vi "SRV_Sensor View Tab GUI.vi"(10 "SRV In":refnum<k5>, 11 "Sensors Config File Path":path) -> (0 "error out":errorcluster)   [LabVIEW 2009]
doc: "A Producer-Consumer two-loop state machine template. This template uses the LPD Command Queues to drive its execution.\n\nThere are several advantages such as:\n- convenient error state control\n- the ability to pass data between states/loops/VIs via a variant\n- command history which is extremely valuable in troubleshooting when an error occurs\n\n\nAuthor: Mike Schultz\n\nLogicPD, Inc\nwww.logicpd.com"
uses:
  SRV_Sensor View refs.ctl
  SRV_Sensor Config Cluster.ctl
  SRV_Sensor Analog-Digital.ctl
  SRV_Sensor Sampling Mode.ctl
  SRV_Sensor View Config Cluster.ctl
  SRV_Sensors Names.ctl
  SRV_Sensor PicoC Shared Var Type.ctl
  SRV_Sensor Config-Command Cluster.ctl
  Support/SRV_Command-Data Queue Data Type.ctl
  SRV_Sensor-Value Cluster.ctl
  <vilib>/Utility/error.llb/DialogType.ctl
panel:
  out "Overflow Indicator":bool
  out "# elements in queue":i32
  out "Command":string
  in  "Poll":bool
  in  "Edit_Boolean 32":bool
  out "Boolean 32":bool
  in  "Edit_Boolean 31":bool
  out "Boolean 31":bool
  in  "Edit_Boolean 30":bool
  out "Boolean 30":bool
  in  "Edit_Boolean 29":bool
  out "Boolean 29":bool
  in  "Edit_Boolean 28":bool
  out "Boolean 28":bool
  in  "Edit_Boolean 27":bool
  out "Boolean 27":bool
  in  "Edit_Boolean 26":bool
  out "Boolean 26":bool
  in  "Edit_Boolean 25":bool
  out "Boolean 25":bool
  in  "Edit_Boolean 24":bool
  out "Boolean 24":bool
  in  "Edit_Boolean 23":bool
  out "Boolean 23":bool
  in  "Edit_Boolean 22":bool
  out "Boolean 22":bool
  in  "Edit_Boolean 21":bool
  out "Boolean 21":bool
  in  "Edit_Boolean 20":bool
  out "Boolean 20":bool
  in  "Edit_Boolean 19":bool
  out "Boolean 19":bool
  in  "Edit_Boolean 18":bool
  out "Boolean 18":bool
  in  "Edit_Boolean 17":bool
  out "Boolean 17":bool
  in  "Edit_Boolean 16":bool
  out "Boolean 16":bool
  in  "Edit_Boolean 15":bool
  out "Boolean 15":bool
  in  "Edit_Boolean 14":bool
  out "Boolean 14":bool
  in  "Edit_Boolean 13":bool
  out "Boolean 13":bool
  in  "Edit_Boolean 12":bool
  out "Boolean 12":bool
  in  "Edit_Boolean 11":bool
  out "Boolean 11":bool
  in  "Edit_Boolean 10":bool
  out "Boolean 10":bool
  in  "Edit_Boolean 09":bool
  out "Boolean 09":bool
  in  "Edit_Boolean 08":bool
  out "Boolean 08":bool
  in  "Edit_Boolean 07":bool
  out "Boolean 07":bool
  in  "Edit_Boolean 06":bool
  out "Boolean 06":bool
  in  "Edit_Boolean 05":bool
  out "Boolean 05":bool
  in  "Edit_Boolean 04":bool
  out "Boolean 04":bool
  in  "Edit_Boolean 03":bool
  out "Boolean 03":bool
  in  "Edit_Boolean 02":bool
  out "Boolean 02":bool
  in  "Edit_Boolean 01":bool
  out "Boolean 01":bool
  in  "Edit_Numeric 08":bool
  out "Numeric 08":dbl
  in  "Edit_Numeric 07":bool
  out "Numeric 07":dbl
  in  "Edit_Numeric 06":bool
  out "Numeric 06":dbl
  in  "Edit_Numeric 05":bool
  out "Numeric 05":dbl
  in  "Edit_Numeric 04":bool
  out "Numeric 04":dbl
  in  "Edit_Numeric 03":bool
  out "Numeric 03":dbl
  in  "Edit_Numeric 02":bool
  out "Numeric 02":dbl
  in  "Edit_Numeric 01":bool
  out "Numeric 01":dbl
  in  "Edit_Meter 04":bool
  out "Meter 04":dbl(knob) scale=-1.0..0.0
  in  "Edit_Meter 03":bool
  out "Meter 03":dbl(knob) scale=-1.0..0.0
  in  "Edit_Meter 02":bool
  out "Meter 02":dbl(knob) caption="6" scale=-1.0..0.0
  in  "Edit_Meter 01":bool
  out "Meter 01":dbl(knob) caption="5" scale=-1.0..0.0
  in  "Edit_Gauge 04":bool
  out "Gauge 04":dbl(knob) caption="4" scale=-1.0..0.0
  in  "Edit_Gauge 03":bool
  out "Gauge 03":dbl(knob) caption="3" scale=-1.0..0.0
  in  "Edit_Gauge 02":bool
  out "Gauge 02":dbl(knob) caption="2" scale=-1.0..0.0
  in  "Edit_Gauge 01":bool
  out "Gauge 01":dbl(knob) caption="1" scale=-1.0..0.0 scale format="%#.3g"
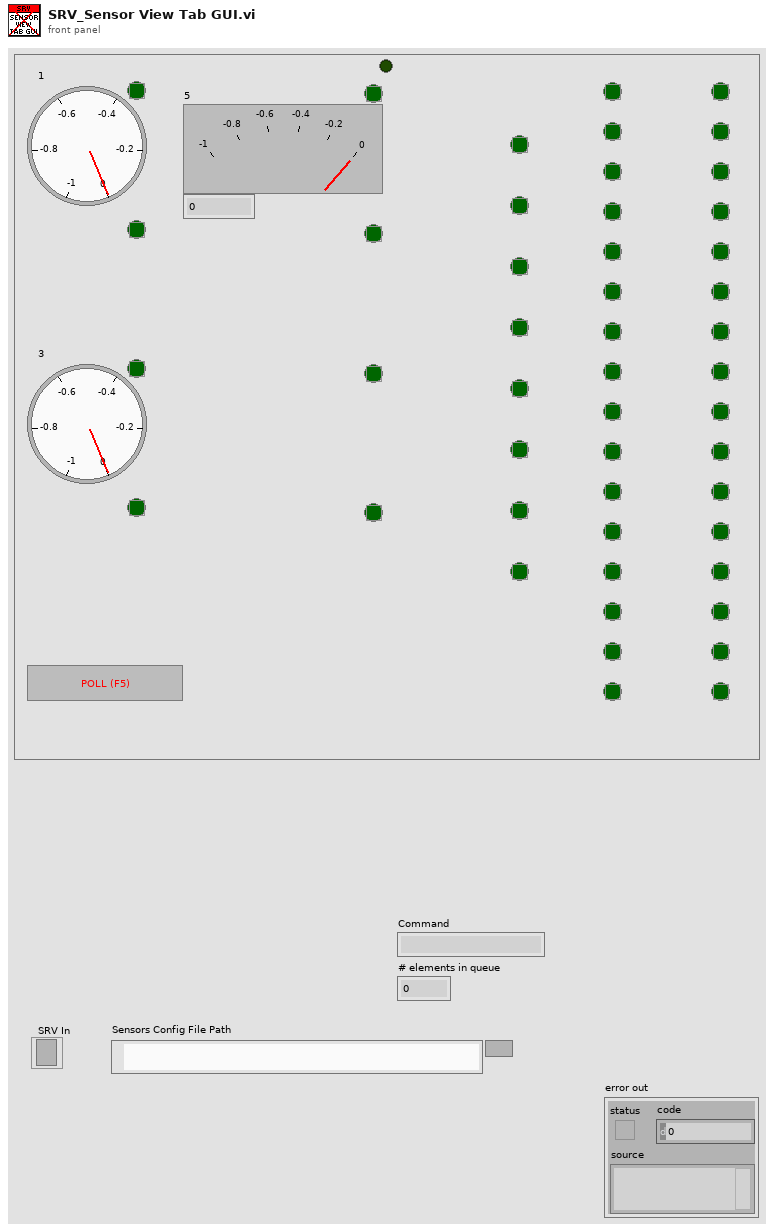
[diagram p1: front panel]
types:
  T1 = typedef "SRV_Command-Data Queue Data Type.ctl" = cluster{"Command":string, "Data":variant}
  T2 = typedef "SRV_Sensor View refs.ctl" = cluster{"Knob refs":refnum<vi>[], "Numeric refs":refnum<vi>[], "Boolean refs":refnum<vi>[]}
  T3 = typedef "SRV_Sensor Config Cluster.ctl" = cluster{"Name":string, "A/D":T4, "I2C Address":u8, "Register":u8, "Channel":u8, "Digital Mask":u8, "Units":string, "Sampling Mode":T5, "Sample Period (ms)":u32, "Formula":string, "Sensor View Config":T6, "Active":bool, "PicoC Shared Var Type":T8, "Index":u8, "Stream Multiple?":bool, "Index End":u8}
  T4 = typedef "SRV_Sensor Analog-Digital.ctl" = enum16{"Analog", "Digital", "RCMx1 Analog", "PicoC Shared"}
  T5 = typedef "SRV_Sensor Sampling Mode.ctl" = enum16{"Polled", "Streaming"}
  T6 = typedef "SRV_Sensor View Config Cluster.ctl" = cluster{"Sensor Name":T7, "Minimum":dbl, "Maximum":dbl}
  T7 = typedef "SRV_Sensors Names.ctl" = enum16{"Gauge 01", "Gauge 02", "Gauge 03", "Gauge 04", "Meter 01", "Meter 02", "Meter 03", "Meter 04", "Numeric 01", "Numeric 02", "Numeric 03", "Numeric 04", "Numeric 05", "Numeric 06", "Numeric 07", "Numeric 08", "Boolean 01", "Boolean 02", "Boolean 03", "Boolean 04", "Boolean 05", "Boolean 06", "Boolean 07", "Boolean 08", "Boolean 09", "Boolean 10", "Boolean 11", "Boolean 12", "Boolean 13", "Boolean 14", "Boolean 15", "Boolean 16", "Boolean 17", "Boolean 18", "Boolean 19", "Boolean 20", "Boolean 21", "Boolean 22", "Boolean 23", "Boolean 24", "Boolean 25", "Boolean 26", "Boolean 27", "Boolean 28", "Boolean 29", "Boolean 30", "Boolean 31", "Boolean 32"}
  T8 = typedef "SRV_Sensor PicoC Shared Var Type.ctl" = enum16{"String", "Integer", "Float"}
  T9 = typedef "SRV_Sensor Config-Command Cluster.ctl" = cluster{"Sensor Config":T3, "Command":string, "Constant Command":string}
  T10 = cluster{"user event":refnum<user-event>, "Version":string, "Sensor View refs":T2, "This VI ref":refnum<vi>, "Sensors Config File Path":path, "Sensors Config":T3[], "SRV ref":refnum<k5>, "Streaming Cfg-Cmds":T9[], "Polled Cfg-Cmds":T9[], "Off Cfg-Cmds":T9[], "Streaming Constant Commands":string[], "Polled Constant Commands":string[]}
  T11 = typedef "SRV_Sensor-Value Cluster.ctl" = cluster{"Sensor Name":T7, "Value":dbl}
  T12 = typedef "DialogType.ctl" = u16
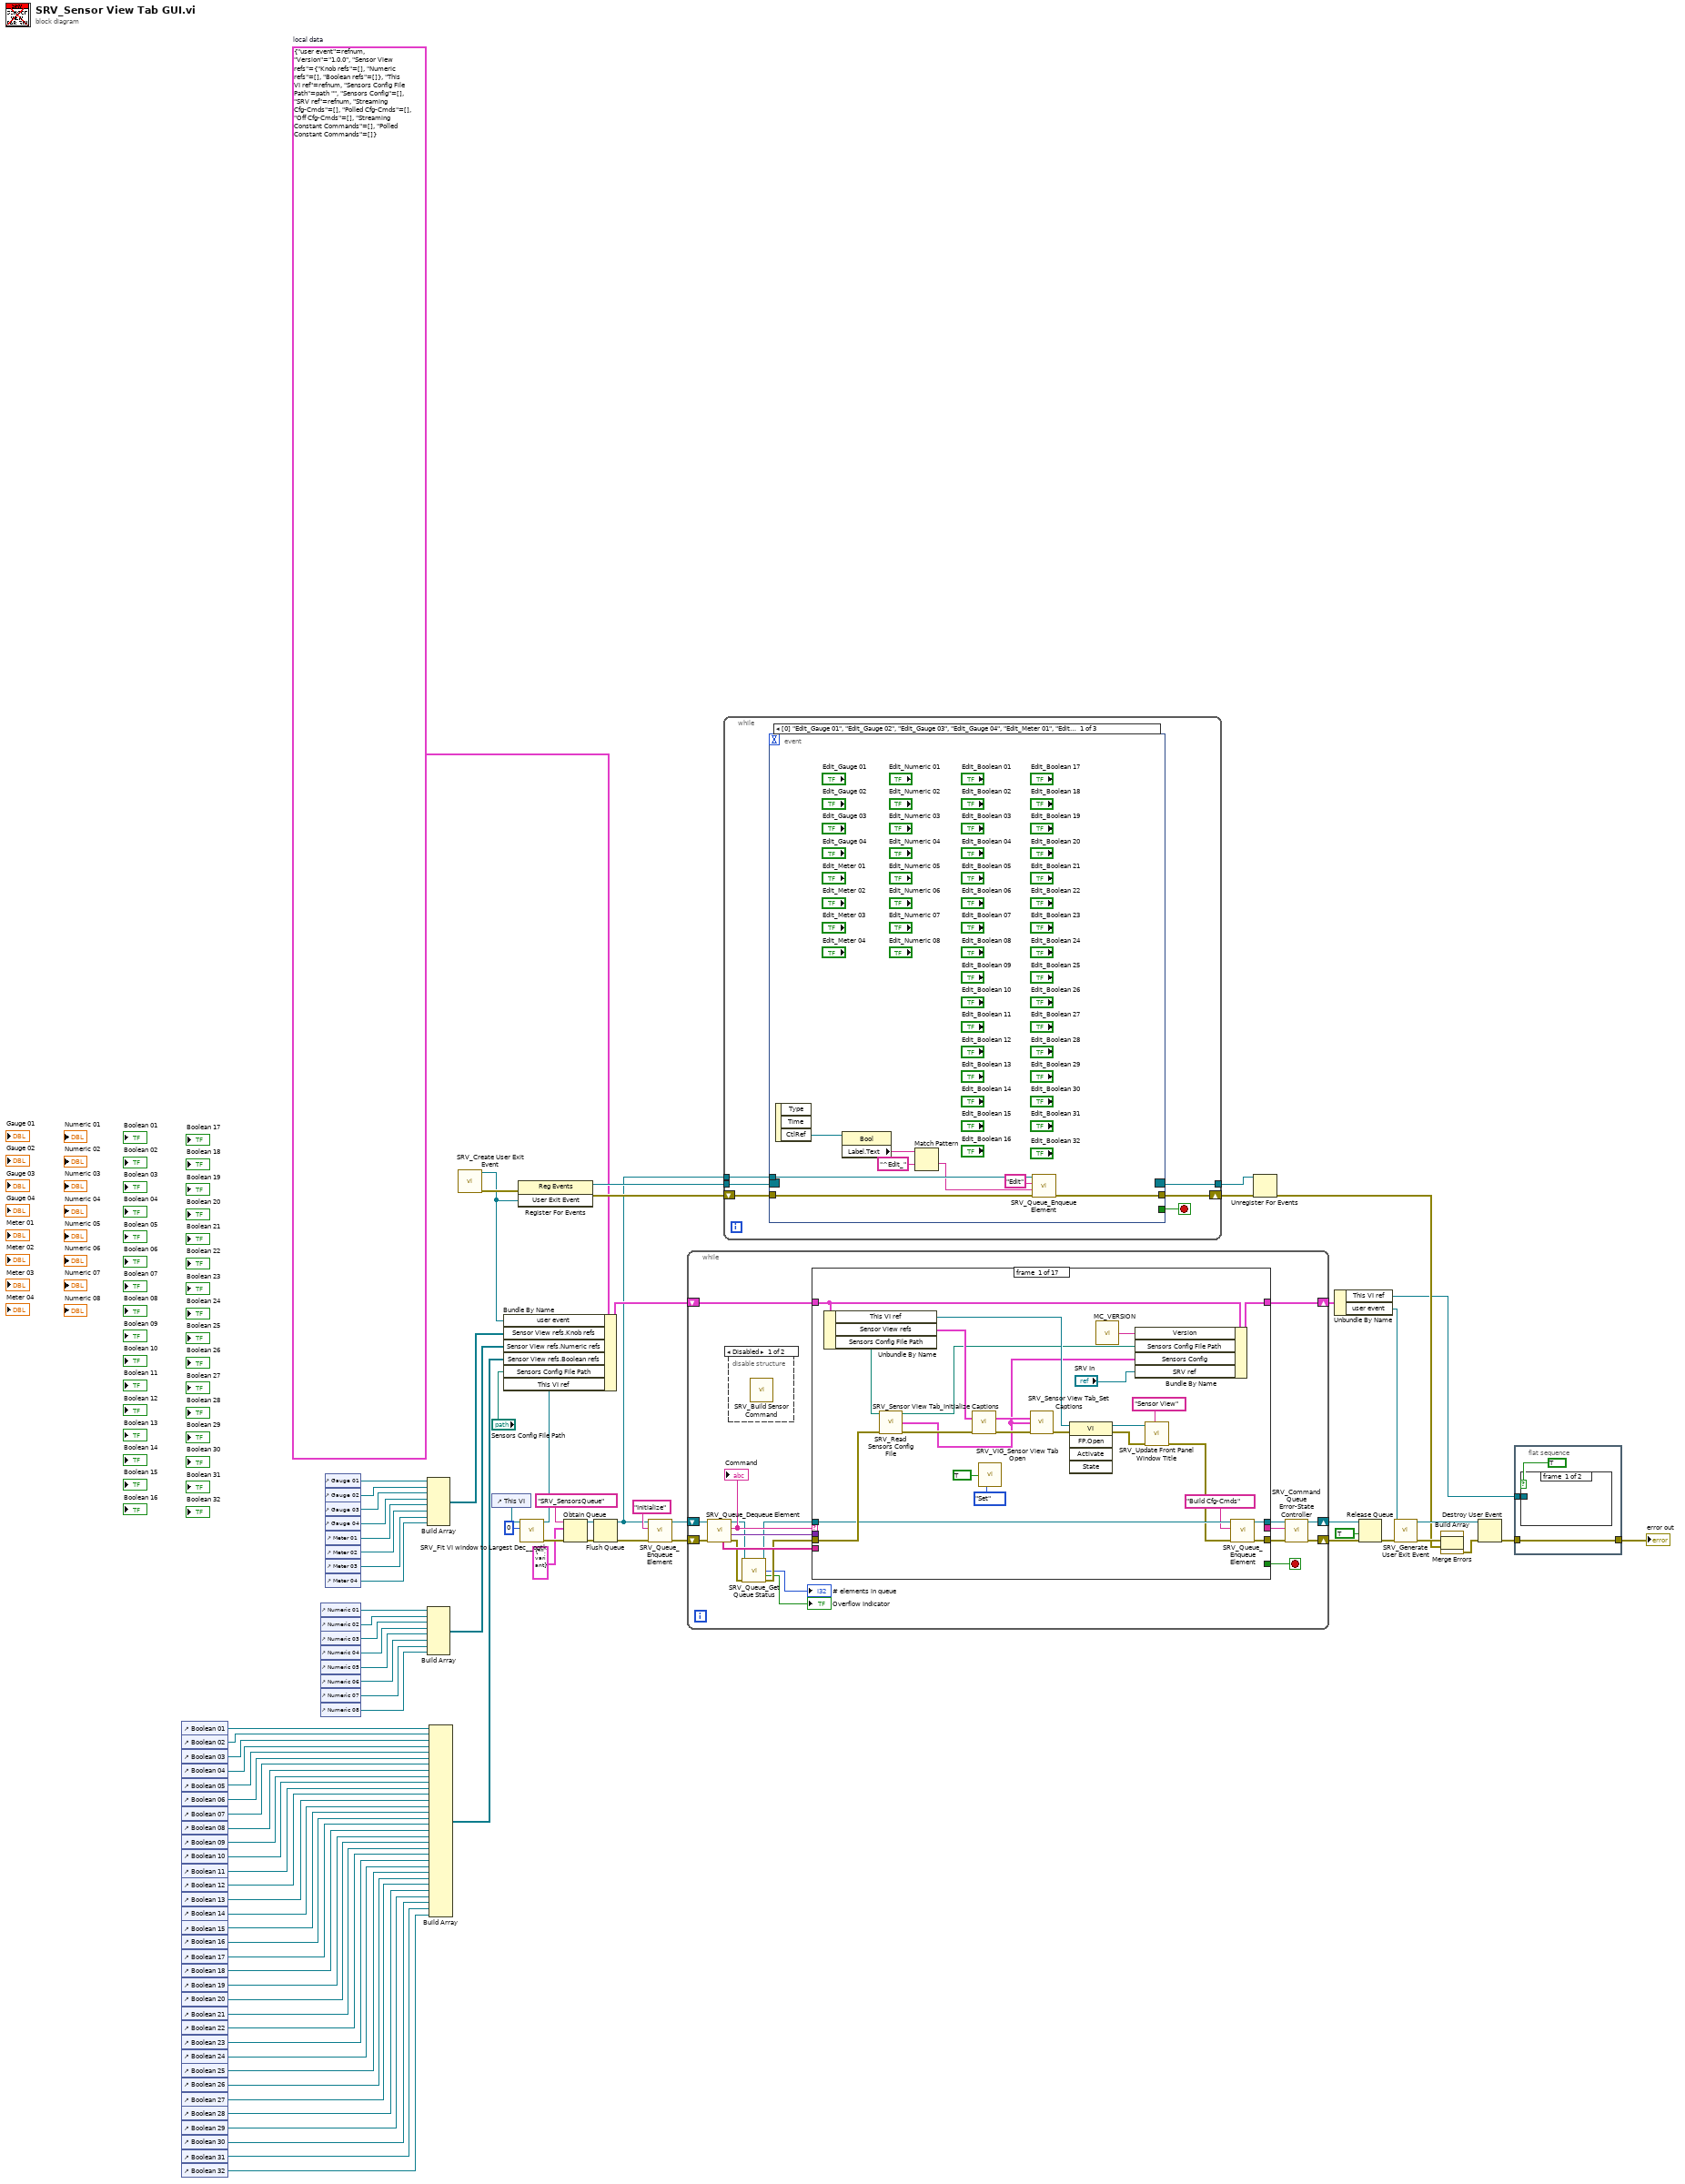
[diagram p0: block diagram]
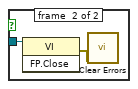
[diagram p2: hidden frame]
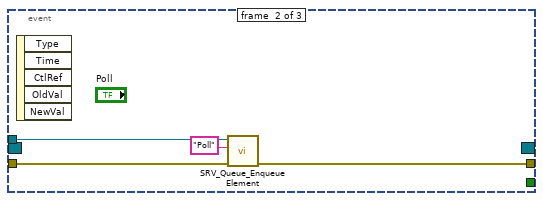
[diagram p3: hidden frame]
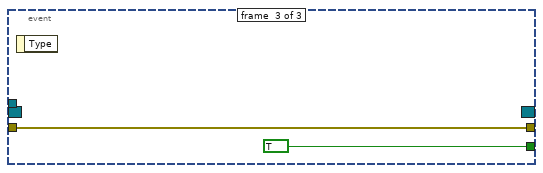
[diagram p4: hidden frame]
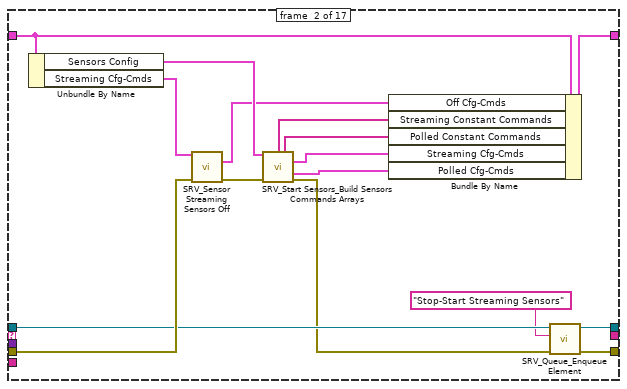
[diagram p6: hidden frame]
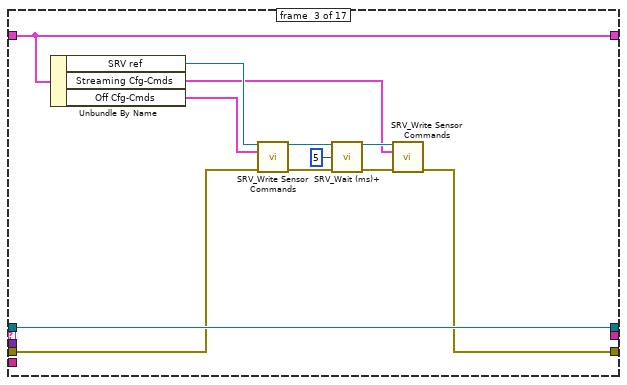
[diagram p7: hidden frame]
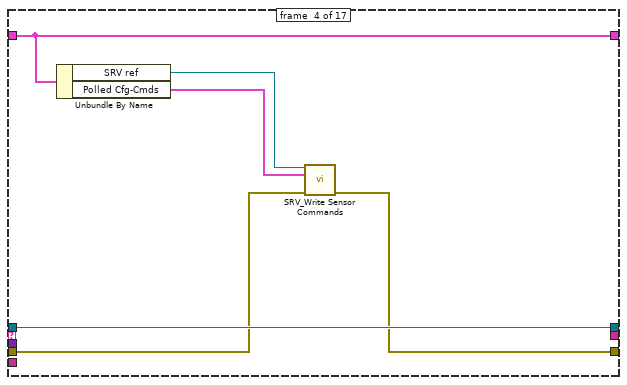
[diagram p8: hidden frame]
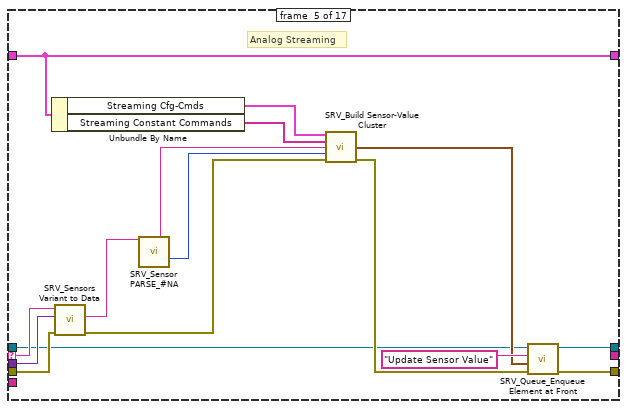
[diagram p9: hidden frame]
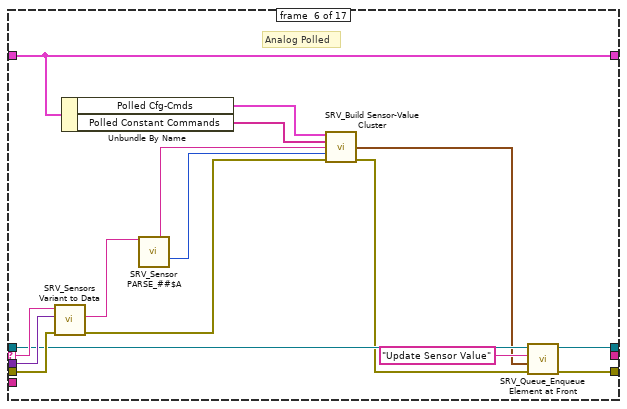
[diagram p10: hidden frame]
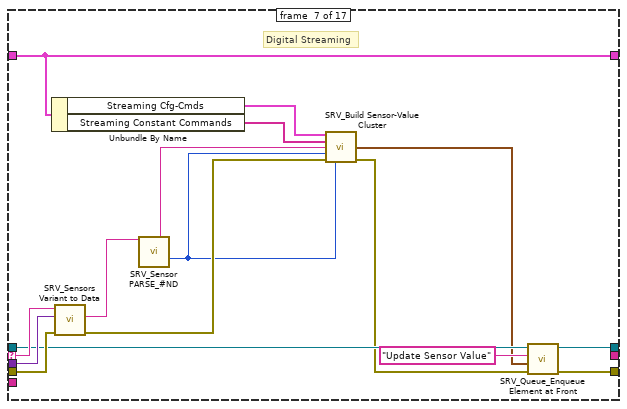
[diagram p11: hidden frame]
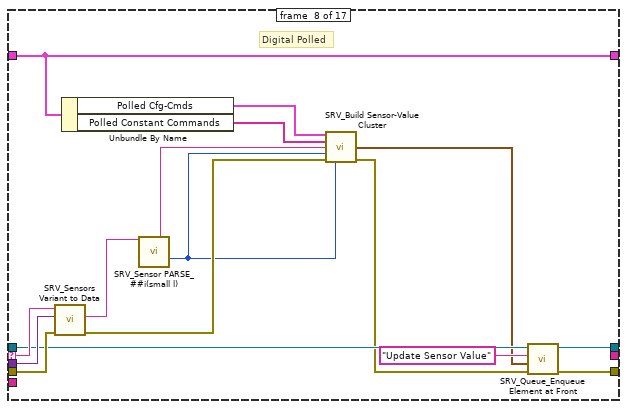
[diagram p12: hidden frame]
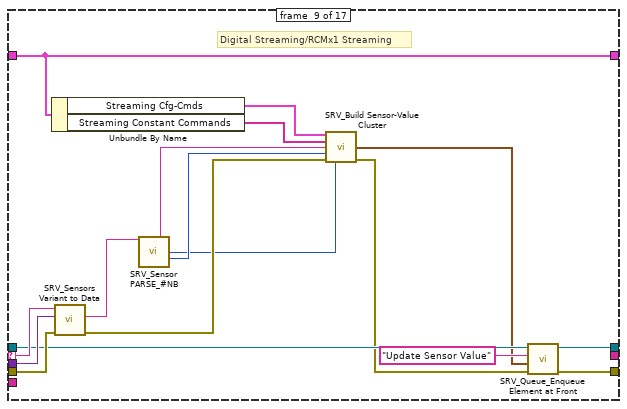
[diagram p13: hidden frame]
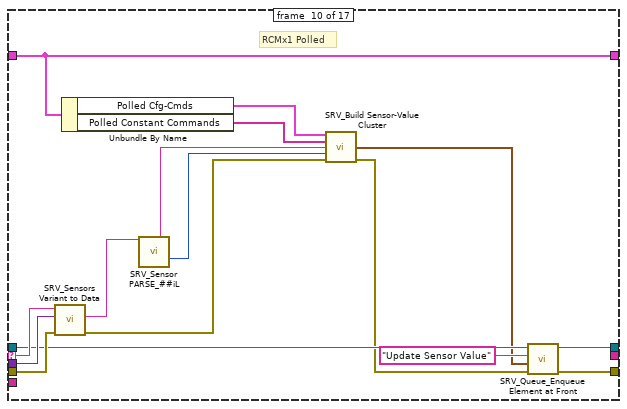
[diagram p14: hidden frame]
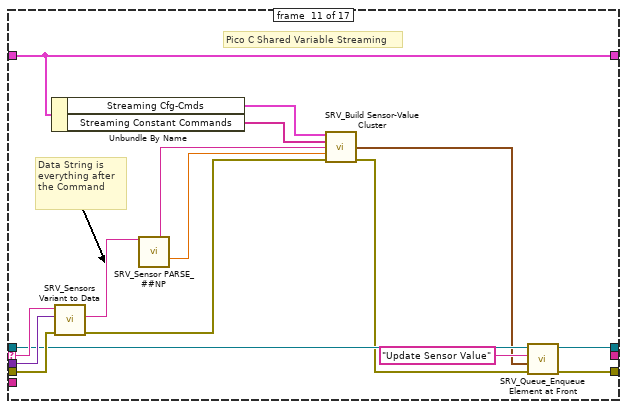
[diagram p15: hidden frame]
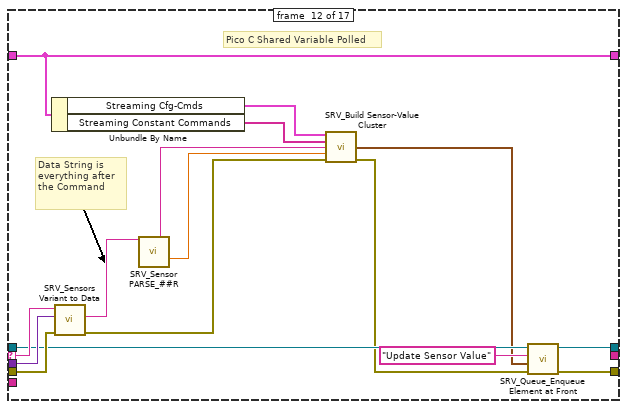
[diagram p16: hidden frame]
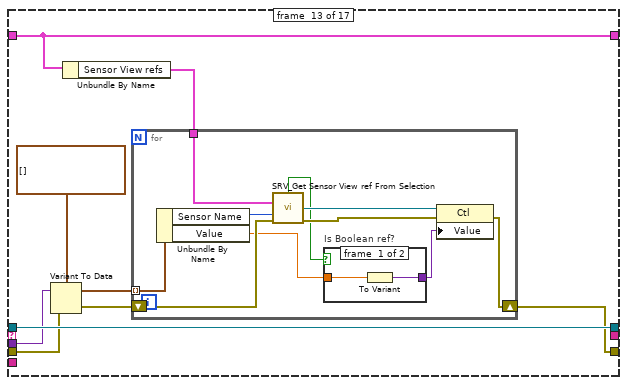
[diagram p17: hidden frame]
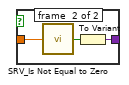
[diagram p18: hidden frame]
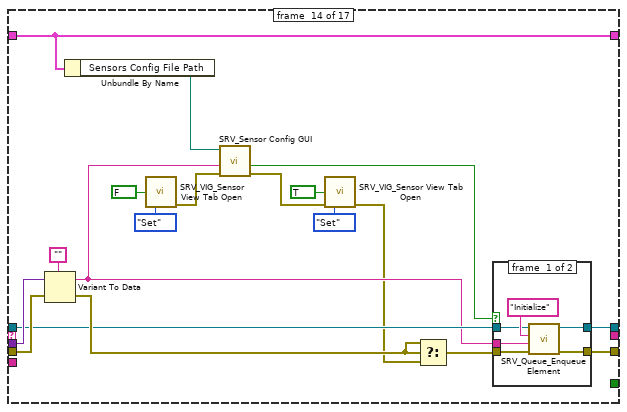
[diagram p19: hidden frame]
diagram:
  w81 = T10 {"user event"=refnum, "Version"="1.0.0", "Sensor View refs"={"Knob refs"=[], "Numeric refs"=[], "Boolean refs"=[]}, "This VI ref"=refnum, "Sensors Config File Path"=path "", "Sensors Config"=[], "SRV ref"=refnum, "Streaming Cfg-Cmds"=[], "Polled Cfg-Cmds"=[], "Off Cfg-Cmds"=[], "Streaming Constant Commands"=[], "Polled Constant Commands"=[]}  # local data
  n1 = control-ref of="Boolean 01"() -> (w48:refnum<vi>)
  n2 = control-ref of="Boolean 02"() -> (w47:refnum<vi>)
  n3 = control-ref of="Boolean 03"() -> (w46:refnum<vi>)
  n4 = control-ref of="Boolean 04"() -> (w45:refnum<vi>)
  n5 = control-ref of="Boolean 05"() -> (w44:refnum<vi>)
  n6 = control-ref of="Boolean 06"() -> (w43:refnum<vi>)
  n7 = control-ref of="Boolean 07"() -> (w42:refnum<vi>)
  n8 = control-ref of="Boolean 08"() -> (w41:refnum<vi>)
  n9 = control-ref of="Boolean 09"() -> (w40:refnum<vi>)
  n10 = control-ref of="Boolean 10"() -> (w39:refnum<vi>)
  n11 = control-ref of="Boolean 11"() -> (w38:refnum<vi>)
  n12 = control-ref of="Boolean 12"() -> (w37:refnum<vi>)
  n13 = control-ref of="Boolean 13"() -> (w36:refnum<vi>)
  n14 = control-ref of="Boolean 14"() -> (w35:refnum<vi>)
  n15 = control-ref of="Boolean 15"() -> (w34:refnum<vi>)
  n16 = control-ref of="Boolean 16"() -> (w33:refnum<vi>)
  n17 = control-ref of="Boolean 17"() -> (w32:refnum<vi>)
  n18 = control-ref of="Boolean 18"() -> (w31:refnum<vi>)
  n19 = control-ref of="Boolean 19"() -> (w30:refnum<vi>)
  n20 = control-ref of="Boolean 20"() -> (w29:refnum<vi>)
  n21 = control-ref of="Boolean 21"() -> (w28:refnum<vi>)
  n22 = control-ref of="Boolean 22"() -> (w27:refnum<vi>)
  n23 = control-ref of="Boolean 23"() -> (w26:refnum<vi>)
  n24 = control-ref of="Boolean 24"() -> (w25:refnum<vi>)
  n25 = control-ref of="Boolean 25"() -> (w24:refnum<vi>)
  n26 = control-ref of="Boolean 26"() -> (w23:refnum<vi>)
  n27 = control-ref of="Boolean 27"() -> (w22:refnum<vi>)
  n28 = control-ref of="Boolean 28"() -> (w21:refnum<vi>)
  n29 = control-ref of="Boolean 29"() -> (w20:refnum<vi>)
  n30 = control-ref of="Boolean 30"() -> (w19:refnum<vi>)
  n31 = control-ref of="Boolean 31"() -> (w18:refnum<vi>)
  n32 = control-ref of="Boolean 32"() -> (w17:refnum<vi>)
  n33 = control-ref of="Numeric 01"() -> (w56:refnum<vi>)
  n34 = control-ref of="Numeric 02"() -> (w55:refnum<vi>)
  n35 = control-ref of="Numeric 03"() -> (w54:refnum<vi>)
  n36 = control-ref of="Numeric 04"() -> (w53:refnum<vi>)
  n37 = control-ref of="Numeric 05"() -> (w52:refnum<vi>)
  n38 = control-ref of="Numeric 06"() -> (w51:refnum<vi>)
  n39 = control-ref of="Numeric 07"() -> (w50:refnum<vi>)
  n40 = control-ref of="Numeric 08"() -> (w49:refnum<vi>)
  n41 = control-ref of="Gauge 01"() -> (w64:refnum<vi>)
  n42 = control-ref of="Gauge 02"() -> (w63:refnum<vi>)
  n43 = control-ref of="Gauge 03"() -> (w62:refnum<vi>)
  n44 = control-ref of="Gauge 04"() -> (w61:refnum<vi>)
  n45 = control-ref of="Meter 01"() -> (w60:refnum<vi>)
  n46 = control-ref of="Meter 02"() -> (w59:refnum<vi>)
  n47 = control-ref of="Meter 03"() -> (w58:refnum<vi>)
  n48 = control-ref of="Meter 04"() -> (w57:refnum<vi>)
  n49 = Build Array(w64, w63, w62, w61, w60, w59, w58, w57) -> (w11:refnum<vi>[])
  n50 = Build Array(w56, w55, w54, w53, w52, w51, w50, w49) -> (w12:refnum<vi>[])
  n51 = Build Array(w48, w47, w46, w45, w44, w43, w42, w41, w40, w39, w38, w37, w36, w35, w34, w33, w32, w31, w30, w29, w28, w27, w26, w25, w24, w23, w22, w21, w20, w19, w18, w17) -> (w13:refnum<vi>[])
  n52 = call "SRV_Create User Exit Event.vi"() -> ("error out"=w72:errorcluster, "User Exit Event"=w71:refnum<user-event>)  [unwired: 10 in]
  n53 = control-ref of="This VI"() -> (w2:refnum<vi>)
  n54 = register-events(error in=w72, w71) -> (reference out=w87:refnum<event-registration>, error out=w86:errorcluster)  [unwired: 1 in]
  n55 = call "SRV_Fit VI window to Largest Dec__ogtk.vi"("border spacing (2 px)"=0, "VI Ref (calling VI)"=w2) -> ("error out"=w67:errorcluster, "dup VI Ref"=w10:refnum<vi>)  [unwired: 4 in]
  n56 = Bundle By Name(cluster=w81, "user event"=w71, "Sensor View refs.Knob refs"=w11, "Sensor View refs.Numeric refs"=w12, "Sensor View refs.Boolean refs"=w13, "Sensors Config File Path"="Sensors Config File Path", "This VI ref"=w10) -> (w80:T10)
  n57 = Obtain Queue(name (unnamed)="SRV_SensorsQueue", element data type=T1 {"Command"="", "Data"=variant} ("Queue Data Type"), error in (no error)=w67) -> (queue out=w4:refnum<queue>, error out=w6:errorcluster)  [unwired: 2 in, 1 out]
  n58 = Flush Queue(queue=w4, error in (no error)=w6) -> (queue out=w3:refnum<queue>, error out=w5:errorcluster)  [unwired: 1 out]
  n59 = call "SRV_Queue_Enqueue Element.vi"("error in (no error)"=w5, "Command"="Initialize", "Command-Data Queue"=w3) -> ("error out"=w65:errorcluster, "Command-Data Queue out"=w68:refnum<queue>)  [unwired: 6 in, 1 out]
  n60 = while {
    shift-right: [w102] -> w83
    shift-left: w65 -> [w106]
    shift-right: [w100] -> w82
    shift-left: w68 -> [w105]
    shift-right: [w94] -> w79
    shift-left: w80 -> [w95]
    stop <- w96 stop-if-true
    n61 = call "SRV_Queue_Dequeue Element.vi"("error in (no error)"=w106, "Command-Data Queue"=w105) -> ("error out"=w93:errorcluster, "Data"=w99:variant, "Command"=w104:string, "Command-Data Queue out"=w91:refnum<queue>, "Command History"=w98:string[])  [unwired: 4 in, 1 out]
    "Command" <- w104
    n62 = disable-structure shown="Disabled" {
      frame #0 {
        n63 = call "SRV_Build Sensor Command.vi"() -> ()  [unwired: 9 in, 7 out]
      }
      frame #1 {
      }
    }
    n64 = call "SRV_Queue_Get Queue Status.vi"("Command-Data Queue"=w91, "error in (no error)"=w93) -> ("Command-Data Queue out"=w90:refnum<queue>, "# elements in queue"=→"# elements in queue":i32, "Overflow Indicator"=→"Overflow Indicator":bool, "error out"=w92:errorcluster)  [unwired: 10 in]
    n65 = case shown="\"Initialize\"" w104 {
      selector: w104 -> [_ _ _ _ w178 w194 w210 w226 w243 w259 w275 w291 _ _ w348 _ _]
      tunnel: w92 -> [w129 w140 w155 w159 w165 w193 w209 w225 w242 w258 w274 w290 w300 w335 w346 w355 w362]
      tunnel: [w116 w135 w150 w158 w169 w182 w199 w215 w232 w247 w263 w279 w294 w328 w345 w352 w361] -> w103
      tunnel: w90 -> [w118 w137 w156 w163 w164 w185 w202 w218 w235 w250 w266 w282 w301 w326 w350 w359 w372]
      tunnel: [w117 w136 w156 w163 w171 w184 w201 w217 w234 w249 w265 w281 w301 w327 w350 w359 w372] -> w101
      tunnel: w99 -> [_ _ _ _ w179 w195 w211 w227 w244 w260 w276 w292 w299 w333 _ _ _]
      tunnel: w98 -> [_ _ _ _ _ _ _ _ _ _ _ _ _ _ _ w358 _]
      tunnel: [_ _ _ _ _ _ _ _ _ _ _ _ _ _ _ "Exit" ("Error Command") _] -> w97
      tunnel: [_ _ _ _ _ _ _ _ _ _ _ _ _ _ _ _ TRUE] -> w96
      tunnel: w95 -> [w127 w145 w157 w162 w176 w191 w207 w223 w240 w256 w272 w288 w298 w331 w347 w356 w368]
      tunnel: [w130 w144 w157 w162 w176 w191 w207 w223 w240 w256 w272 w288 w298 w331 w347 w356 w368] -> w94
      frame #0 {
        n66 = Unbundle By Name(w127) -> ("This VI ref"=w123:refnum<vi>, "Sensor View refs"=w126:T2, "Sensors Config File Path"=w120:path)
        n67 = call "SRV_Read Sensors Config File.vi"("Sensors Config File Path"=w120, "error in (no error)"=w129) -> ("Sensors Config File Path out"=w121:path, "Sensors Config"=w119:T3[], "error out"=w128:errorcluster)  [unwired: 10 in, 1 out]
        n68 = call "SRV_Sensor View Tab_Initialize Captions.vi"("Sensor View refs"=w126, "error in (no error)"=w128) -> ("Sensor View refs dup"=w124:T2, "error out"=w125:errorcluster)  [unwired: 12 in]
        n69 = call "SRV_VIG_Sensor View Tab Open.vi"("Sensor View Tab Open"=TRUE, "Method (Get)"=enum16{"Get", "Set"}."Set") -> ()  [unwired: 12 in, 2 out]
        n70 = call "SRV_Sensor View Tab_Set Captions.vi"("Sensor View refs"=w124, "Sensors Config"=w119, "error in (no error)"=w125) -> ("error out"=w122:errorcluster)  [unwired: 11 in, 1 out]
        n71 = invoke class="VI" method="FP.Open"(reference=w123, error in=w122) -> (reference out=w111:refnum<vi>, error out=w112:errorcluster)  [unwired: 3 in, 3 out]
        n72 = call "MC_VERSION.vi"() -> ("MC Version"=w113:string)
        n73 = Bundle By Name(cluster=w127, "Version"=w113, "Sensors Config File Path"=w121, "Sensors Config"=w119, "SRV ref"="SRV In") -> (w130:T10)
        n74 = call "SRV_Update Front Panel Window Title.vi"("Window Title Override String"="Sensor View", "error in (no error)"=w112, "VI ref"=w111) -> ("error out"=w110:errorcluster)  [unwired: 7 in, 1 out]
        n75 = call "SRV_Queue_Enqueue Element.vi"("error in (no error)"=w110, "Command"="Build Cfg-Cmds", "Command-Data Queue"=w118) -> ("error out"=w116:errorcluster, "Command-Data Queue out"=w117:refnum<queue>)  [unwired: 6 in, 1 out]
      }
      frame #1 {
        n76 = Unbundle By Name(w145) -> ("Sensors Config"=w146:T3[], "Streaming Cfg-Cmds"=w141:T9[])
        n77 = call "SRV_Sensor Streaming Sensors Off.vi"("Previous Streaming Cfg-Cmds"=w141, "error in (no error)"=w140) -> ("Streaming Cfg-Cmds OFF"=w138:T9[], "error out"=w139:errorcluster)  [unwired: 12 in]
        n78 = call "SRV_Start Sensors_Build Sensors Commands Arrays.vi"("Sensors Config"=w146, "error in (no error)"=w139) -> ("Streaming Constant Commands"=w132:string[], "Polled Constant Commands"=w131:string[], "Active Streaming Cfg-Commands"=w143:T9[], "Active Polled Cfg-Commands"=w142:T9[], "error out"=w134:errorcluster)  [unwired: 9 in]
        n79 = Bundle By Name(cluster=w145, "Off Cfg-Cmds"=w138, "Streaming Constant Commands"=w132, "Polled Constant Commands"=w131, "Streaming Cfg-Cmds"=w143, "Polled Cfg-Cmds"=w142) -> (w144:T10)
        n80 = call "SRV_Queue_Enqueue Element.vi"("error in (no error)"=w134, "Command"="Stop-Start Streaming Sensors", "Command-Data Queue"=w137) -> ("error out"=w135:errorcluster, "Command-Data Queue out"=w136:refnum<queue>)  [unwired: 6 in, 1 out]
      }
      frame #2 {
        n81 = Unbundle By Name(w157) -> ("SRV ref"=w154:refnum<k5>, "Streaming Cfg-Cmds"=w151:T9[], "Off Cfg-Cmds"=w153:T9[])
        n82 = call "SRV_Write Sensor Commands.vi"("SRV In"=w154, "Sensor Cfg-Commands"=w153, "error in (no error)"=w155) -> ("SRV out"=w152:refnum<k5>, "error out"=w149:errorcluster)  [unwired: 11 in]
        n83 = call "SRV_Wait (ms)+.vi"("milliseconds to wait"=u32 5, "error in (no error)"=w149) -> ("error out"=w148:errorcluster)  [unwired: 12 in, 1 out]
        n84 = call "SRV_Write Sensor Commands.vi"("SRV In"=w152, "Sensor Cfg-Commands"=w151, "error in (no error)"=w148) -> ("error out"=w150:errorcluster)  [unwired: 11 in, 1 out]
      }
      frame #3 {
        n85 = Unbundle By Name(w162) -> ("SRV ref"=w160:refnum<k5>, "Polled Cfg-Cmds"=w161:T9[])
        n86 = call "SRV_Write Sensor Commands.vi"("SRV In"=w160, "Sensor Cfg-Commands"=w161, "error in (no error)"=w159) -> ("error out"=w158:errorcluster)  [unwired: 11 in, 1 out]
      }
      frame #4 {
        # "Analog Streaming"
        n87 = Unbundle By Name(w176) -> ("Streaming Cfg-Cmds"=w175:T9[], "Streaming Constant Commands"=w174:string[])
        n88 = call "SRV_Sensors Variant to Data.vi"("error in (no error)"=w165, "Data"=w179, "Command"=w178) -> ("error out"=w166:errorcluster, "Data String"=w177:string)  [unwired: 7 in]
        n89 = call "SRV_Sensor PARSE_#NA.vi"("Return Data"=w177) -> ("Constant Command"=w173:string, "Value"=w172:u16)  [unwired: 13 in]
        n90 = call "SRV_Build Sensor-Value Cluster.vi"("Cfg-Cmds"=w175, "Constant Commands"=w174, "Constant Command"=w173, "Value"=w172, "error in (no error)"=w166) -> ("Array of Sensor-Value Cluster"=w167:T11[], "error out"=w170:errorcluster)  [unwired: 9 in]
        n91 = call "SRV_Queue_Enqueue Element at Front.vi"("error in (no error)"=w170, "Data"=w167, "Command"="Update Sensor Value", "Command-Data Queue"=w164) -> ("error out"=w169:errorcluster, "Command-Data Queue out"=w171:refnum<queue>)  [unwired: 5 in, 1 out]
      }
      frame #5 {
        # "Analog Polled"
        n92 = call "SRV_Sensors Variant to Data.vi"("error in (no error)"=w193, "Data"=w195, "Command"=w194) -> ("error out"=w186:errorcluster, "Data String"=w192:string)  [unwired: 7 in]
        n93 = Unbundle By Name(w191) -> ("Polled Cfg-Cmds"=w190:T9[], "Polled Constant Commands"=w189:string[])
        n94 = call "SRV_Sensor PARSE_##$A.vi"("Return Data"=w192) -> ("Constant Command"=w188:string, "Value"=w187:u16)  [unwired: 13 in]
        n95 = call "SRV_Build Sensor-Value Cluster.vi"("Cfg-Cmds"=w190, "Constant Commands"=w189, "Constant Command"=w188, "Value"=w187, "error in (no error)"=w186) -> ("Array of Sensor-Value Cluster"=w180:T11[], "error out"=w183:errorcluster)  [unwired: 9 in]
        n96 = call "SRV_Queue_Enqueue Element at Front.vi"("error in (no error)"=w183, "Data"=w180, "Command"="Update Sensor Value", "Command-Data Queue"=w185) -> ("error out"=w182:errorcluster, "Command-Data Queue out"=w184:refnum<queue>)  [unwired: 5 in, 1 out]
      }
      frame #6 {
        # "Digital Streaming"
        n97 = Unbundle By Name(w207) -> ("Streaming Cfg-Cmds"=w206:T9[], "Streaming Constant Commands"=w205:string[])
        n98 = call "SRV_Sensors Variant to Data.vi"("error in (no error)"=w209, "Data"=w211, "Command"=w210) -> ("error out"=w203:errorcluster, "Data String"=w208:string)  [unwired: 7 in]
        n99 = call "SRV_Sensor PARSE_#ND.vi"("Return Data"=w208) -> ("Constant Command"=w204:string, "Value"=w196:u8)  [unwired: 13 in]
        n100 = call "SRV_Build Sensor-Value Cluster.vi"("Cfg-Cmds"=w206, "Constant Commands"=w205, "Constant Command"=w204, "Value"=w196, "error in (no error)"=w203, "Value (U8)"=w196) -> ("Array of Sensor-Value Cluster"=w197:T11[], "error out"=w200:errorcluster)  [unwired: 8 in]
        n101 = call "SRV_Queue_Enqueue Element at Front.vi"("error in (no error)"=w200, "Data"=w197, "Command"="Update Sensor Value", "Command-Data Queue"=w202) -> ("error out"=w199:errorcluster, "Command-Data Queue out"=w201:refnum<queue>)  [unwired: 5 in, 1 out]
      }
      frame #7 {
        # "Digital Polled"
        n102 = call "SRV_Sensors Variant to Data.vi"("error in (no error)"=w225, "Data"=w227, "Command"=w226) -> ("error out"=w219:errorcluster, "Data String"=w224:string)  [unwired: 7 in]
        n103 = Unbundle By Name(w223) -> ("Polled Cfg-Cmds"=w222:T9[], "Polled Constant Commands"=w221:string[])
        n104 = call "SRV_Sensor PARSE_##i(small l).vi"("Return Data"=w224) -> ("Constant Command"=w220:string, "Value"=w212:u8)  [unwired: 13 in]
        n105 = call "SRV_Build Sensor-Value Cluster.vi"("Cfg-Cmds"=w222, "Constant Commands"=w221, "Constant Command"=w220, "Value"=w212, "error in (no error)"=w219, "Value (U8)"=w212) -> ("Array of Sensor-Value Cluster"=w213:T11[], "error out"=w216:errorcluster)  [unwired: 8 in]
        n106 = call "SRV_Queue_Enqueue Element at Front.vi"("error in (no error)"=w216, "Data"=w213, "Command"="Update Sensor Value", "Command-Data Queue"=w218) -> ("error out"=w215:errorcluster, "Command-Data Queue out"=w217:refnum<queue>)  [unwired: 5 in, 1 out]
      }
      frame #8 {
        # "Digital Streaming/RCMx1 Streaming"
        n107 = Unbundle By Name(w240) -> ("Streaming Cfg-Cmds"=w239:T9[], "Streaming Constant Commands"=w238:string[])
        n108 = call "SRV_Sensors Variant to Data.vi"("error in (no error)"=w242, "Data"=w244, "Command"=w243) -> ("error out"=w236:errorcluster, "Data String"=w241:string)  [unwired: 7 in]
        n109 = call "SRV_Sensor PARSE_#NB.vi"("Return Data"=w241) -> ("Constant Command"=w237:string, "Value (U8)"=w228:u8, "Value"=w229:u16)  [unwired: 12 in]
        n110 = call "SRV_Build Sensor-Value Cluster.vi"("Cfg-Cmds"=w239, "Constant Commands"=w238, "Constant Command"=w237, "Value"=w229, "error in (no error)"=w236, "Value (U8)"=w228) -> ("Array of Sensor-Value Cluster"=w230:T11[], "error out"=w233:errorcluster)  [unwired: 8 in]
        n111 = call "SRV_Queue_Enqueue Element at Front.vi"("error in (no error)"=w233, "Data"=w230, "Command"="Update Sensor Value", "Command-Data Queue"=w235) -> ("error out"=w232:errorcluster, "Command-Data Queue out"=w234:refnum<queue>)  [unwired: 5 in, 1 out]
      }
      frame #9 {
        # "RCMx1 Polled"
        n112 = call "SRV_Sensors Variant to Data.vi"("error in (no error)"=w258, "Data"=w260, "Command"=w259) -> ("error out"=w251:errorcluster, "Data String"=w257:string)  [unwired: 7 in]
        n113 = Unbundle By Name(w256) -> ("Polled Cfg-Cmds"=w255:T9[], "Polled Constant Commands"=w254:string[])
        n114 = call "SRV_Sensor PARSE_##iL.vi"("Return Data"=w257) -> ("Constant Command"=w253:string, "Value"=w252:u16)  [unwired: 13 in]
        n115 = call "SRV_Build Sensor-Value Cluster.vi"("Cfg-Cmds"=w255, "Constant Commands"=w254, "Constant Command"=w253, "Value"=w252, "error in (no error)"=w251) -> ("Array of Sensor-Value Cluster"=w245:T11[], "error out"=w248:errorcluster)  [unwired: 9 in]
        n116 = call "SRV_Queue_Enqueue Element at Front.vi"("error in (no error)"=w248, "Data"=w245, "Command"="Update Sensor Value", "Command-Data Queue"=w250) -> ("error out"=w247:errorcluster, "Command-Data Queue out"=w249:refnum<queue>)  [unwired: 5 in, 1 out]
      }
      frame #10 {
        # "Data String is everything after the Command"
        # "Pico C Shared Variable Streaming"
        n117 = Unbundle By Name(w272) -> ("Streaming Cfg-Cmds"=w271:T9[], "Streaming Constant Commands"=w270:string[])
        n118 = call "SRV_Sensors Variant to Data.vi"("error in (no error)"=w274, "Data"=w276, "Command"=w275) -> ("error out"=w267:errorcluster, "Data String"=w273:string)  [unwired: 7 in]
        n119 = call "SRV_Sensor PARSE_##NP.vi"("Return Data"=w273) -> ("Constant Command"=w269:string, "Value"=w268:dbl)  [unwired: 13 in]
        n120 = call "SRV_Build Sensor-Value Cluster.vi"("Cfg-Cmds"=w271, "Constant Commands"=w270, "Constant Command"=w269, "Value"=w268, "error in (no error)"=w267) -> ("Array of Sensor-Value Cluster"=w261:T11[], "error out"=w264:errorcluster)  [unwired: 9 in]
        n121 = call "SRV_Queue_Enqueue Element at Front.vi"("error in (no error)"=w264, "Data"=w261, "Command"="Update Sensor Value", "Command-Data Queue"=w266) -> ("error out"=w263:errorcluster, "Command-Data Queue out"=w265:refnum<queue>)  [unwired: 5 in, 1 out]
      }
      frame #11 {
        # "Data String is everything after the Command"
        # "Pico C Shared Variable Polled"
        n122 = Unbundle By Name(w288) -> ("Streaming Cfg-Cmds"=w287:T9[], "Streaming Constant Commands"=w286:string[])
        n123 = call "SRV_Sensors Variant to Data.vi"("error in (no error)"=w290, "Data"=w292, "Command"=w291) -> ("error out"=w283:errorcluster, "Data String"=w289:string)  [unwired: 7 in]
        n124 = call "SRV_Sensor PARSE_##R.vi"("Return Data"=w289) -> ("Constant Command"=w285:string, "Value"=w284:dbl)  [unwired: 13 in]
        n125 = call "SRV_Build Sensor-Value Cluster.vi"("Cfg-Cmds"=w287, "Constant Commands"=w286, "Constant Command"=w285, "Value"=w284, "error in (no error)"=w283) -> ("Array of Sensor-Value Cluster"=w277:T11[], "error out"=w280:errorcluster)  [unwired: 9 in]
        n126 = call "SRV_Queue_Enqueue Element at Front.vi"("error in (no error)"=w280, "Data"=w277, "Command"="Update Sensor Value", "Command-Data Queue"=w282) -> ("error out"=w279:errorcluster, "Command-Data Queue out"=w281:refnum<queue>)  [unwired: 5 in, 1 out]
      }
      frame #12 {
        n127 = Variant To Data(error in=w300, Variant=w299, type=T11[] [] ("Array of Sensor-Value Cluster")) -> (error out=w295:errorcluster, data=w296:T11[])
        n128 = Unbundle By Name(w298) -> ("Sensor View refs"=w297:T2)
        n129 = for {
          tunnel: w297 -> [w311]
          tunnel: w296 -> [w310] mode=indexing
          shift-right: [w305] -> w294
          shift-left: w295 -> [w308]
          n130 = Unbundle By Name(w310) -> ("Sensor Name"=w309:T7, "Value"=w303:dbl)
          n131 = call "SRV_Get Sensor View ref From Selection.vi"("Sensor View refs"=w311, "Sensor View"=w309, "error in (no error)"=w308) -> ("Boolean ref?"=w304:bool, "Selected ref"=w307:refnum<vi>, "error out"=w306:errorcluster)  [unwired: 8 in, 2 out]
          n132 = case "Is Boolean ref?" shown="True" w304 {
            tunnel: w303 -> [w313 w316]
            tunnel: [w312 w314] -> w302
            frame #0 {
              n133 = To Variant(anything=w313) -> (Variant=w312:variant)
            }
            frame #1 {
              n134 = call "SRV_Is Not Equal to Zero.vi"("Numeric (DBL)"=w316) -> ("Not Zero"=w315:bool)  [unwired: 14 in]
              n135 = To Variant(anything=w315) -> (Variant=w314:variant)
            }
          }
          n136 = property class="Ctl"(reference=w307, error in=w306, "Value"=w302) -> (error out=w305:errorcluster)  [unwired: 1 out]
        }
      }
      frame #13 {
        n137 = Variant To Data(error in=w335, Variant=w333, type="") -> (error out=w332:errorcluster, data=w324:string)
        n138 = Unbundle By Name(w331) -> ("Sensors Config File Path"=w330:path)
        n139 = call "SRV_VIG_Sensor View Tab Open.vi"("Sensor View Tab Open"=FALSE, "Method (Get)"=enum16{"Get", "Set"}."Set") -> ("error out"=w317:errorcluster)  [unwired: 12 in, 1 out]
        n140 = call "SRV_Sensor Config GUI.vi"("error in (no error)"=w317, "Sensor to Edit"=w324, "Sensors Config File Path in"=w330) -> ("error out"=w319:errorcluster, "Cancelled?"=w325:bool)  [unwired: 6 in, 1 out]
        n141 = call "SRV_VIG_Sensor View Tab Open.vi"("Sensor View Tab Open"=TRUE, "error in (no error)"=w319, "Method (Get)"=enum16{"Get", "Set"}."Set") -> ("error out"=w318:errorcluster)  [unwired: 11 in, 1 out]
        n142 = Select(t=w332, s=w332, f=w318) -> (s? t:f=w329:errorcluster)
        n143 = case shown="False" w325 {
          tunnel: w329 -> [w340 w342]
          tunnel: [w339 w342] -> w328
          tunnel: [w338 w343] -> w327
          tunnel: w326 -> [w337 w343]
          tunnel: w324 -> [w336 _]
          frame #0 {
            n144 = call "SRV_Queue_Enqueue Element.vi"("error in (no error)"=w340, "Data"=w336, "Command"="Initialize", "Command-Data Queue"=w337) -> ("error out"=w339:errorcluster, "Command-Data Queue out"=w338:refnum<queue>)  [unwired: 5 in, 1 out]
          }
          frame #1 {
          }
        }
      }
      frame #14 {
        # "generates an error with a useful message when an undefined state is requested"
        n145 = Format Into String(format string="Developer Error: the case \"%s\" is undefined.", w348) -> (resulting string=w344:string)  [unwired: 2 in, 1 out]
        n146 = call "SRV_Generate Error.vi"("Message"=w344, "error in (no error)"=w346) -> ("error out"=w345:errorcluster)  [unwired: 13 in]
      }
      frame #15 {
        w351 = T12 1 items=["no dialog", "OK message", "continue or stop message", "OK message + warnings", "continue/stop + warnings"] ("type of dialog (OK msg:1)")
        # "Use Default If Unwired because in the other cases empty string is the same as wiring \"Error\" in the Error-State Controller VI"
        # "append the recent command history to the error souce string"
        n147 = call "SRV_Format Command History String.vi"("Command History"=w358) -> ("Command History String"=w354:string)  [unwired: 14 in]
        n148 = call "SRV_Append to New Error Source String.vi"("Message String to append"=w354, "Error In (no error)"=w355) -> ("error out"=w353:errorcluster)  [unwired: 13 in]
        n149 = call <vilib>:"General Error Handler.vi"("type of dialog (OK msg:1)"=w351, "error in (no error)"=w353) -> ("error out"=w352:errorcluster)  [unwired: 9 in, 4 out]
      }
      frame #16 {
        n150 = call "SRV_VIG_Sensor View Tab Open.vi"("Sensor View Tab Open"=FALSE, "Method (Get)"=enum16{"Get", "Set"}."Set") -> ("error out"=w363:errorcluster)  [unwired: 12 in, 1 out]
        n151 = Unbundle By Name(w368) -> ("SRV ref"=w365:refnum<k5>, "Streaming Cfg-Cmds"=w367:T9[])
        n152 = call "SRV_Sensor Streaming Sensors Off.vi"("Previous Streaming Cfg-Cmds"=w367, "error in (no error)"=w363) -> ("Streaming Cfg-Cmds OFF"=w364:T9[], "error out"=w366:errorcluster)  [unwired: 12 in]
        n153 = call "SRV_Write Sensor Commands.vi"("SRV In"=w365, "Sensor Cfg-Commands"=w364, "error in (no error)"=w366) -> ("error out"=w360:errorcluster)  [unwired: 11 in, 1 out]
        n154 = Select(t=w362, s=w362, f=w360) -> (s? t:f=w361:errorcluster)
      }
    }
    n155 = call "SRV_Command Queue Error-State Controller.vi"("error in (no error)"=w103, "Error Command"=w97, "Command-Data Queue"=w101) -> ("error out"=w102:errorcluster, "Command-Data Queue out"=w100:refnum<queue>)  [unwired: 7 in]
  }
  n156 = while {
    shift-right: [w377] -> w84
    shift-left: w86 -> [w378]
    tunnel: w3 -> [w376]
    tunnel: w87 -> [w375]
    tunnel: [w374] -> w85
    stop <- w373 stop-if-true
    n157 = event shown="[0] \"Edit_Gauge 01\", \"Edit_Gauge 02\", \"Edit_Gauge 03\", \"Edit_Gauge 04\", \"Edit_Meter 01\", \"Edit_Meter 02\", \"Edit_Meter 03\", \"Edit_Meter 04\", \"Edit_Numeric 01\", \"Edit_Numeric 02\", \"Edit_Numeric 03\", \"Edit_Numeric 04\", \"Edit_Numeric 05\", \"Edit_Numeric 06\", \"Edit_Numeric 07\", \"Edit_Numeric 08\", \"Edit_Boolean 01\", \"Edit_Boolean 02\", \"Edit_Boolean 03\", \"Edit_Boolean 04\", \"Edit_Boolean 05\", \"Edit_Boolean 06\", \"Edit_Boolean 07\", \"Edit_Boolean 08\", \"Edit_Boolean 09\", \"Edit_Boolean 10\", \"Edit_Boolean 11\", \"Edit_Boolean 12\", \"Edit_Boolean 13\", \"Edit_Boolean 14\", \"Edit_Boolean 15\", \"Edit_Boolean 16\", \"Edit_Boolean 17\", \"Edit_Boolean 18\", \"Edit_Boolean 19\", \"Edit_Boolean 20\", \"Edit_Boolean 21\", \"Edit_Boolean 22\", \"Edit_Boolean 23\", \"Edit_Boolean 24\", \"Edit_Boolean 25\", \"Edit_Boolean 26\", \"Edit_Boolean 27\", \"Edit_Boolean 28\", \"Edit_Boolean 29\", \"Edit_Boolean 30\", \"Edit_Boolean 31\", \"Edit_Boolean 32\": Value Change" {
      selector: w375 -> [_ _ _]
      dyn-events: [_ _ _] -> w374
      timeout: _ -> [_ _ _]
      tunnel: w378 -> [w386 w388 w392]
      tunnel: [w385 w389 w392] -> w377
      tunnel: w376 -> [w384 w387 _]
      tunnel: [_ _ TRUE] -> w373
      event #0 {
        n158 = event-data() -> ("CtlRef"=w383:refnum<vi>)  [unwired: 1 in, 2 out]
        n159 = property class="Bool"(reference=w383) -> ("Label.Text"=w382:string)  [unwired: 1 in, 2 out]
        n160 = Match Pattern(string=w382, regular expression="^Edit_") -> (after substring=w379:string)  [unwired: 1 in, 3 out]
        n161 = call "SRV_Queue_Enqueue Element.vi"("error in (no error)"=w386, "Data"=w379, "Command"="Edit", "Command-Data Queue"=w384) -> ("error out"=w385:errorcluster)  [unwired: 5 in, 2 out]
      }
      event #1 {
        n162 = event-data() -> ()  [unwired: 1 in, 5 out]
        n163 = call "SRV_Queue_Enqueue Element.vi"("error in (no error)"=w388, "Command"="Poll", "Command-Data Queue"=w387) -> ("error out"=w389:errorcluster)  [unwired: 6 in, 2 out]
      }
      event #2 {
        n164 = event-data() -> ()  [unwired: 1 in, 1 out]
      }
    }
  }
  n165 = Unregister For Events(event registration refnum=w85, error in=w84) -> (error out=w74:errorcluster)
  n166 = Unbundle By Name(w79) -> ("This VI ref"=w14:refnum<vi>, "user event"=w78:refnum<user-event>)
  n167 = Release Queue(queue=w82, force destroy? (F)=TRUE, error in (no error)=w83) -> (error out=w77:errorcluster)  [unwired: 2 out]
  n168 = call "SRV_Generate User Exit Event.vi"("error in (no error)"=w77, "User Exit Event"=w78) -> ("error out"=w75:errorcluster, "User Exit Event out"=w76:refnum<user-event>)  [unwired: 8 in]
  n169 = Build Array(w75, w74) -> (w70:errorcluster[])
  n170 = call <vilib>:"Merge Errors.vi"("error array in"=w70) -> ("error out"=w73:errorcluster)  [unwired: 6 in]
  n171 = Destroy User Event(user event=w76, error in=w73) -> (error out=w16:errorcluster)
  n172 = flat-sequence {
    tunnel: w16 -> [w395]
    tunnel: [w395] -> w15
    tunnel: w14 -> [w394]
    frame #0 {
      n173 = case shown="True" TRUE {
        tunnel: w394 -> [_ w397]
        frame #0 {
        }
        frame #1 {
          n174 = invoke class="VI" method="FP.Close"(reference=w397) -> (error out=w396:errorcluster)  [unwired: 2 in, 2 out]
          n175 = call <vilib>:"Clear Errors.vi"("error in (no error)"=w396) -> ()  [unwired: 6 in, 1 out]
        }
      }
    }
  }
  "error out" <- w15
